vi "HiTech-Color-Senser_Read.vi"(7 "Color Mode":u16(ring) items=["RGB", "HSL", "HSV", "HSI", "CIE L*a*b*", "CIE XYZ"], 8 "Error In":errorcluster, 11 "HiTechnicColorSensorV2 Ref In":cluster{"I2C Ref Out":T2}) -> (0 "Error Out":errorcluster, 2 "All Info":T1, 3 "HiTechnicColorSensorV2 Ref Out":cluster{"I2C Ref Out":T2})   [LabVIEW 2019]
uses:
  <vilib>/myRIO/Instrument Drivers/Onboard IO/I2C/typedefs/I2C Reference.ctl
  <vilib>/myRIO/Common/Instrument Driver Framework/Utilities/typedefs/myRIO Generic Hardware Reference.ctl
  <vilib>/myRIO/Common/Instrument Driver Framework/Utilities/typedefs/Hardware Version Enum.ctl
  <vilib>/myRIO/Common/Instrument Driver Framework/Utilities/typedefs/myRIO v1.0 Reference.ctl
  <vilib>/myRIO/Common/Instrument Driver Framework/Utilities/typedefs/Generic FPGA Reference.ctl
  <vilib>/myRIO/Common/Instrument Driver Framework/myRIO v1.0/I2C/typedefs/I2C Channels Enum.ctl
  <vilib>/myRIO/Instrument Drivers/Onboard IO/I2C/typedefs/I2C Configuration.ctl
  <vilib>/myRIO/Instrument Drivers/Onboard IO/I2C/typedefs/I2C Transfer Rate.ctl
  <vilib>/Utility/error.llb/Error Cluster From Error Code.vi
  <vilib>/myRIO/Common/Instrument Driver Framework/myRIO v1.0/I2C/vis/myRIO v1.0 Write I2C.vi
  <vilib>/myRIO/Common/Instrument Driver Framework/myRIO v1.0/I2C/vis/myRIO v1.0 Read I2C.vi
  <vilib>/vision/NI_Vision_Development_Module.lvlib
  <vilib>/myRIO/Instrument Drivers/Onboard IO/I2C/I2C.lvlib
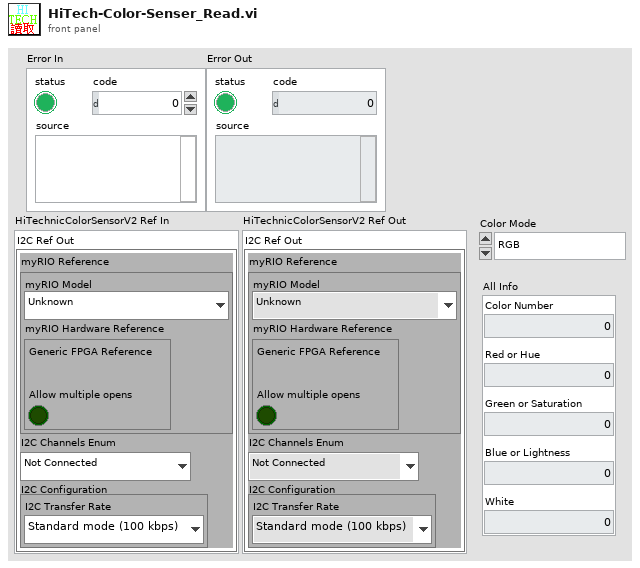
[diagram p1: front panel]
types:
  T1 = cluster{"Color Number":i32, "Red or Hue":i32, "Green or Saturation":i32, "Blue or Lightness":i32, "White":i32}
  T2 = typedef "I2C.lvlib/I2C Reference.ctl" = cluster{"myRIO Reference":T3, "I2C Channels Enum":T7, "I2C Configuration":T8}
  T3 = typedef "myRIO Generic Hardware Reference.ctl" = cluster{"myRIO Model":T4, "myRIO Hardware Reference":T5}
  T4 = typedef "Hardware Version Enum.ctl" = enum16{"Unknown", "myRIO-1900", "myRIO-1950", "roboRIO", "NI ELVIS RIO CM", "ELVIS III"}
  T5 = typedef "myRIO v1.0 Reference.ctl" = cluster{"Generic FPGA Reference":T6, "Allow multiple opens":bool}
  T6 = typedef "Generic FPGA Reference.ctl" = refnum<k20>
  T7 = typedef "I2C Channels Enum.ctl" = enum16{"Not Connected", "A/I2C", "B/I2C", "I2C/I2C"}
  T8 = typedef "I2C.lvlib/I2C Configuration.ctl" = cluster{"I2C Transfer Rate":T9}
  T9 = typedef "I2C.lvlib/I2C Transfer Rate.ctl" = enum16{"Standard mode (100 kbps)", "Fast mode (400 kbps)"}
  T10 = cluster{"Color Number":i32, "Red":i32, "Green":i32, "Blue":i32, "White":i32}
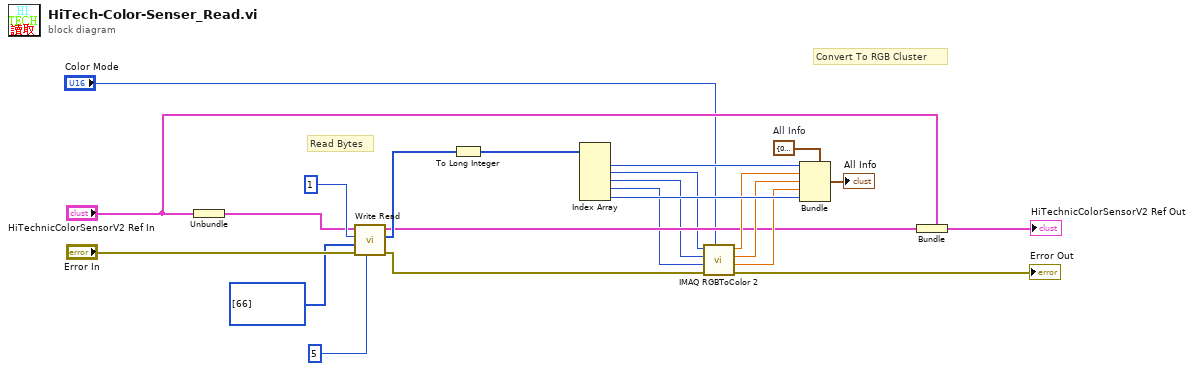
[diagram p0: block diagram]
diagram:
  w11 = T10 {"Color Number"=0, "Red"=0, "Green"=0, "Blue"=0, "White"=0}  # All Info
  # "Read Bytes"
  # "Convert To RGB Cluster"
  n1 = Unbundle("HiTechnicColorSensorV2 Ref In") -> ("I2C Ref Out"=w10:T2)
  n2 = call <vilib>:"Write Read.vi"("Byte Count"=u32 5, "error in (no error)"="Error In", "Bytes to Write"=u8[] [66], "Slave Address (7-bit)"=u8 1, "I2C Ref In"=w10) -> ("error out"=w14:errorcluster, "Bytes Read"=w23:u8[], "I2C Ref Out"=w8:T2)  [unwired: 3 in]
  n3 = To Long Integer(number=w23) -> (32bit integer=w22:i32[])
  n4 = Index Array(array=w22) -> (element #1=w20:i32, element #2=w3:i32, element #3=w2:i32, element #4=w1:i32, element #5=w21:i32)  [unwired: 5 in]
  n5 = call "IMAQ RGBToColor 2"("Color Mode"="Color Mode", "error in (no error)"=w14, "Blue value"=w1, "Green value"=w2, "Red value"=w3) -> ("error out"=→"Error Out":errorcluster, "Blue or Luma or Val or Inten or Z or b*value"=w17:dbl, "Green or Sat or Y or a* value"=w18:dbl, "Red or Hue or X or L* value"=w19:dbl)  [unwired: 3 in]
  n6 = Bundle(cluster=w11, "Color Number"=w20, "Red"=w19, "Green"=w18, "Blue"=w17, "White"=w21) -> (→"All Info":T10)
  n7 = Bundle(cluster="HiTechnicColorSensorV2 Ref In", "I2C Ref Out"=w8) -> (→"HiTechnicColorSensorV2 Ref Out":cluster{"I2C Ref Out":T2})
